vi "Wait for Control Panel Exit.vi"(8 "error in (no error)":errorcluster, 10 "timeout in ms (-1)":i32=-1, 11 "Generic Controller in":refnum<class "Generic Plugin.lvclass">) -> (0 "error out":errorcluster, 2 "Timeout?":bool, 3 "Generic Controller out":refnum<class "Generic Plugin.lvclass">)   [LabVIEW 2020, in "Generic Plugin.lvclass"]
uses:
  Generic Plugin.lvclass
  Generic Plugin.lvclass/Generic Plugin.ctl
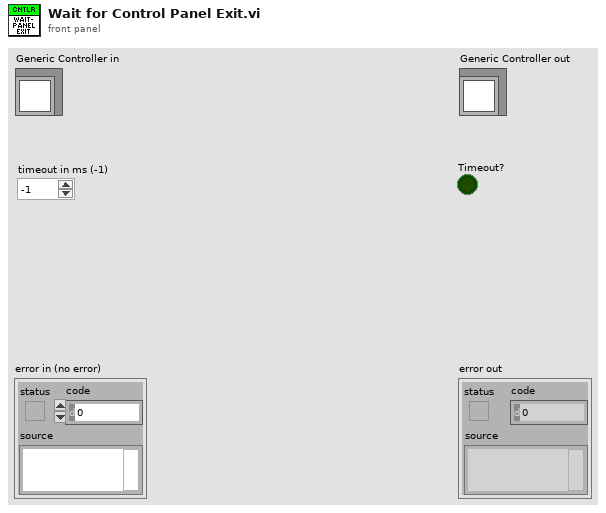
[diagram p1: front panel]
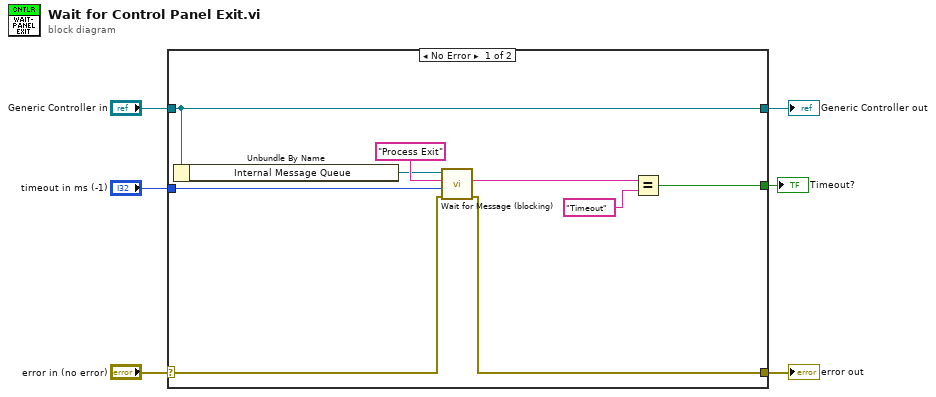
[diagram p0: block diagram]
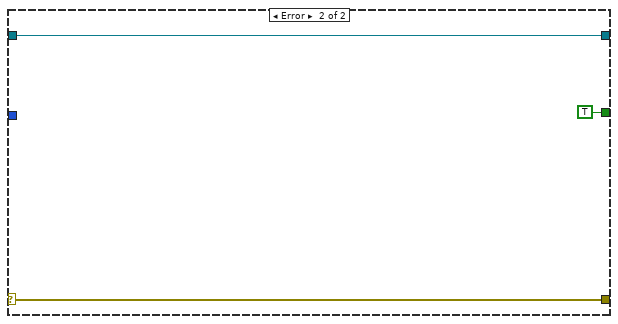
[diagram p2: hidden frame]
diagram:
  n1 = case shown="No Error" "error in (no error)" {
    selector: "error in (no error)" -> [w15 w18]
    tunnel: [w14 w18] -> w5
    tunnel: [w13 w17] -> w3
    tunnel: "Generic Controller in" -> [w13 w17]
    tunnel: "timeout in ms (-1)" -> [w10 _]
    tunnel: [w7 TRUE] -> w1
    frame No Error {
      n2 = Unbundle By Name(w13) -> ("Internal Message Queue"=w11:refnum<queue>)
      n3 = call "Wait for Message (blocking).vi"("error in (no error)"=w15, "timeout in ms (-1)"=w10, "Command"="Process Exit", "Listening queue in"=w11) -> ("error out"=w14:errorcluster, "Message"=w8:string)  [unwired: 4 in, 2 out]
      n4 = Equal?(x=w8, y="Timeout") -> (x = y?=w7:bool)
    }
    frame Error {
    }
  }
  "error out" <- w5
  "Generic Controller out" <- w3
  "Timeout?" <- w1
